vi "GetTime.vi"(1 "日期格式":string="Y-M-D h:m:s") -> (0 "输出":string)   [LabVIEW 2014]
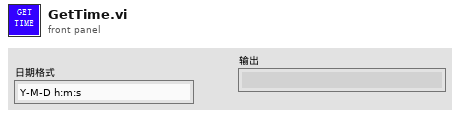
[diagram p1: front panel]
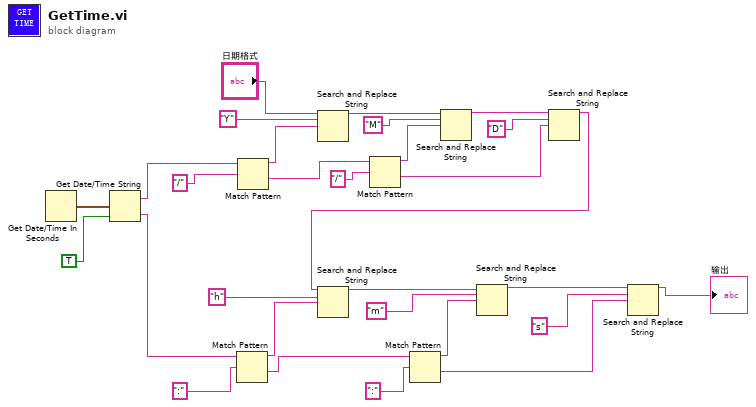
[diagram p0: block diagram]
diagram:
  n1 = Get Date/Time In Seconds() -> (seconds since 1Jan1904=w29:timestamp)
  n2 = Get Date/Time String(seconds (now)=w29, want seconds? (F)=TRUE) -> (date string=w27:string, time string=w14:string)  [unwired: 1 in]
  n3 = Match Pattern(string=w14, regular expression=":") -> (before substring=w12:string, after substring=w8:string)  [unwired: 1 in, 2 out]
  n4 = Match Pattern(string=w27, regular expression="/") -> (before substring=w24:string, after substring=w22:string)  [unwired: 1 in, 2 out]
  n5 = Search and Replace String(input string="日期格式", search string="Y", replace string=w24) -> (result string=w20:string)  [unwired: 5 in, 3 out]
  n6 = Match Pattern(string=w22, regular expression="/") -> (before substring=w19:string, after substring=w17:string)  [unwired: 1 in, 2 out]
  n7 = Match Pattern(string=w8, regular expression=":") -> (before substring=w7:string, after substring=w3:string)  [unwired: 1 in, 2 out]
  n8 = Search and Replace String(input string=w20, search string="M", replace string=w19) -> (result string=w16:string)  [unwired: 5 in, 3 out]
  n9 = Search and Replace String(input string=w16, search string="D", replace string=w17) -> (result string=w10:string)  [unwired: 5 in, 3 out]
  n10 = Search and Replace String(input string=w10, search string="h", replace string=w12) -> (result string=w6:string)  [unwired: 5 in, 3 out]
  n11 = Search and Replace String(input string=w6, search string="m", replace string=w7) -> (result string=w4:string)  [unwired: 5 in, 3 out]
  n12 = Search and Replace String(input string=w4, search string="s", replace string=w3) -> (result string=→"输出":string)  [unwired: 5 in, 3 out]
